vi "SC TCP Check Connection Status.vi"(8 "error in (no error)":errorcluster, 11 "TCP Connection in":refnum<k5>) -> (0 "error out":errorcluster, 2 "Connected":bool, 3 "TCP  Connection out":refnum<k5>)   [LabVIEW 2018]
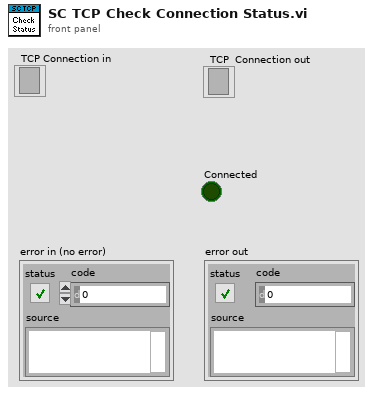
[diagram p1: front panel]
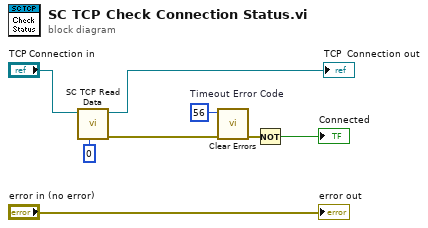
[diagram p0: block diagram]
diagram:
  w3 = 56  # Timeout Error Code
  n1 = call "SC TCP Read Data.vi"("timeout ms (25000)"=0, "TCP  Connection in"="TCP Connection in") -> ("error out"=w5:errorcluster, "TCP  Connection out"=→"TCP  Connection out":refnum<k5>)  [unwired: 7 in, 1 out]
  n2 = call <vilib>:"Clear Errors.vi"("error in (no error)"=w5, "specific error code to clear (0: all)"=w3) -> ("error out"=w8:errorcluster)  [unwired: 4 in, 1 out]
  n3 = Not(x=w8) -> (.not. x?=→"Connected":bool)
  "error out" <- "error in (no error)"
